vi "诊断标定3 - 副本.vi"(8 "CAN端口":u16(ring), 9 "设备索引号":u16(ring), 10 "CAN卡类型":u32(ring)=21) -> ()   [LabVIEW 2013] (continued)
                    }
                  }
                }
              }
            }
          }
          event "DO1": Value Change {
            n2402 = event-data() -> ("NewVal"=w2943:bool)  [unwired: 6 out]
            n2403 = stacked-sequence {
              tunnel: w2943 -> [_ w2956 _]
              frame #0 {
                w2946 = FALSE ("清BUFF")
                n2404 = local write "继电器超时处理"(FALSE ("继电器超时处理")) -> ()
                n2405 = local write "清BUFF"(w2946) -> ()
                n2406 = local write "正级继电器 9"(w2946) -> ()
                n2407 = local write "主从选择"(enum32{"主板", "从板"}."主板" ("主从选择")) -> ()
              }
              frame #1 {
                n2408 = case shown="真" w2956 {
                  selector: w2956 -> [w2971 w2991]
                  tunnel: [w2970 w2990] -> w2955
                  tunnel: [w2958 w2978] -> w2950
                  frame False {
                    w2966 = 256.0 ("y")
                    w2958 = u32 2 ("命令序号")
                    w2970 = u8 192 ("命令")
                    n2409 = local read "动作保持时间"() -> (w2967:dbl)
                    n2410 = Quotient & Remainder(x=w2967, y=w2966) -> (x-y*floor(x/y)=w2959:dbl, floor(x/y)=w2963:dbl)
                    n2411 = Quotient & Remainder(x=w2963, y=w2966) -> (x-y*floor(x/y)=w2960:dbl, floor(x/y)=w2964:dbl)
                    n2412 = Quotient & Remainder(x=w2964, y=w2966) -> (x-y*floor(x/y)=w2961:dbl, floor(x/y)=w2965:dbl)
                    n2413 = local read "设备索引号"() -> (w2975:u16)
                    n2414 = local read "CAN卡类型"() -> (w2976:u32)
                    n2415 = local read "CAN端口"() -> (w2974:u16)
                    n2416 = Boolean To (0,1)(Boolean=w2971) -> (0, 1=w2968:i16)
                    n2417 = Quotient & Remainder(x=w2965, y=w2966) -> (x-y*floor(x/y)=w2962:dbl)  [unwired: 1 out]
                    n2418 = Build Array(i16 1 ("元素"), w2968, w2962, w2961, w2960, w2959, 0.0 ("元素")) -> (w2972:dbl[])
                    n2419 = call "多帧发送机制(EV05).vi"("can卡类型"=w2976, "设备索引号"=w2975, "CAN端口"=w2974, "命令"=w2970, "板号"=u8 0, "命令序号"=w2958, "输入数据"=w2972) -> ()  [unwired: 1 in, 12 out]
                  }
                  frame True {
                    w2986 = 256.0 ("y")
                    w2978 = u32 2 ("命令序号")
                    w2990 = u8 192 ("命令")
                    n2420 = local read "动作保持时间"() -> (w2987:dbl)
                    n2421 = Quotient & Remainder(x=w2987, y=w2986) -> (x-y*floor(x/y)=w2979:dbl, floor(x/y)=w2983:dbl)
                    n2422 = Quotient & Remainder(x=w2983, y=w2986) -> (x-y*floor(x/y)=w2980:dbl, floor(x/y)=w2984:dbl)
                    n2423 = Quotient & Remainder(x=w2984, y=w2986) -> (x-y*floor(x/y)=w2981:dbl, floor(x/y)=w2985:dbl)
                    n2424 = local read "设备索引号"() -> (w2995:u16)
                    n2425 = local read "CAN卡类型"() -> (w2996:u32)
                    n2426 = local read "CAN端口"() -> (w2994:u16)
                    n2427 = Boolean To (0,1)(Boolean=w2991) -> (0, 1=w2988:i16)
                    n2428 = Quotient & Remainder(x=w2985, y=w2986) -> (x-y*floor(x/y)=w2982:dbl)  [unwired: 1 out]
                    n2429 = Build Array(i16 1 ("元素"), w2988, w2982, w2981, w2980, w2979, 0.0 ("元素")) -> (w2992:dbl[])
                    n2430 = call "多帧发送机制(EV05).vi"("can卡类型"=w2996, "设备索引号"=w2995, "CAN端口"=w2994, "命令"=w2990, "板号"=u8 0, "命令序号"=w2978, "输入数据"=w2992) -> ()  [unwired: 1 in, 12 out]
                  }
                }
                n2431 = local write "命令序号"(w2950) -> ()
                n2432 = local write "命令"(w2955) -> ()
                n2433 = local write "控制1"(TRUE ("控制1")) -> ()
                n2434 = local write "写?"(FALSE ("写?")) -> ()
                n2435 = local write "消除"(TRUE ("消除")) -> ()
                n2436 = global write "EV05全局变量1.vi" "流控帧 2"(TRUE ("流控帧 2")) -> ()
                n2437 = global write "EV05全局变量1.vi" "流控帧"(FALSE ("流控帧")) -> ()
              }
              frame #2 {
                n2438 = flat-sequence {
                  tunnel: [w2998] -> w2997
                  tunnel: w2997 -> [w3005]
                  frame #0 {
                    n2439 = while {
                      tunnel: [w2999] -> w2998
                      i -> [w3003]
                      stop <- w3000 stop-if-true
                      n2440 = local read "继电器超时处理"() -> (w2999:bool)
                      n2441 = Greater Or Equal?(x=w3003, y=20) -> (x >= y?=w3001:bool)
                      n2442 = Wait Until Next ms Multiple(millisecond multiple=u32 100 ("毫秒倍数")) -> ()  [unwired: 1 out]
                      n2443 = Or(x=w2999, y=w3001) -> (x .or. y?=w3000:bool)
                    }
                  }
                  frame #1 {
                    n2444 = case shown="假" w3005 {
                      frame False {
                        n2445 = local read "DO1"() -> (w3007:bool)
                        n2446 = Not(x=w3007) -> (.not. x?=w3006:bool)
                        n2447 = local write "DO1"(w3006) -> ()
                        n2448 = One Button Dialog(message="DO控制处理超时" ("消息"), button name ("OK")="是" ("按钮名称（“确定”）")) -> ()  [unwired: 1 out]
                      }
                      frame True {
                      }
                    }
                  }
                }
              }
            }
          }
          event "DO2": Value Change {
            n2449 = event-data() -> ("NewVal"=w3010:bool)  [unwired: 6 out]
            n2450 = stacked-sequence {
              tunnel: w3010 -> [_ w3023 _]
              frame #0 {
                w3013 = FALSE ("清BUFF")
                n2451 = local write "继电器超时处理"(FALSE ("继电器超时处理")) -> ()
                n2452 = local write "主从选择"(enum32{"主板", "从板"}."主板" ("主从选择")) -> ()
                n2453 = local write "清BUFF"(w3013) -> ()
                n2454 = local write "正级继电器 10"(w3013) -> ()
              }
              frame #1 {
                n2455 = case shown="真" w3023 {
                  selector: w3023 -> [w3038 w3058]
                  tunnel: [w3037 w3057] -> w3022
                  tunnel: [w3025 w3045] -> w3017
                  frame False {
                    w3033 = 256.0 ("y")
                    w3025 = u32 2 ("命令序号")
                    w3037 = u8 192 ("命令")
                    n2456 = local read "动作保持时间"() -> (w3034:dbl)
                    n2457 = Quotient & Remainder(x=w3034, y=w3033) -> (x-y*floor(x/y)=w3026:dbl, floor(x/y)=w3030:dbl)
                    n2458 = Quotient & Remainder(x=w3030, y=w3033) -> (x-y*floor(x/y)=w3027:dbl, floor(x/y)=w3031:dbl)
                    n2459 = Quotient & Remainder(x=w3031, y=w3033) -> (x-y*floor(x/y)=w3028:dbl, floor(x/y)=w3032:dbl)
                    n2460 = local read "设备索引号"() -> (w3042:u16)
                    n2461 = local read "CAN卡类型"() -> (w3043:u32)
                    n2462 = local read "CAN端口"() -> (w3041:u16)
                    n2463 = Boolean To (0,1)(Boolean=w3038) -> (0, 1=w3035:i16)
                    n2464 = Quotient & Remainder(x=w3032, y=w3033) -> (x-y*floor(x/y)=w3029:dbl)  [unwired: 1 out]
                    n2465 = Build Array(i16 2 ("元素"), w3035, w3029, w3028, w3027, w3026, 0.0 ("元素")) -> (w3039:dbl[])
                    n2466 = call "多帧发送机制(EV05).vi"("can卡类型"=w3043, "设备索引号"=w3042, "CAN端口"=w3041, "命令"=w3037, "板号"=u8 0, "命令序号"=w3025, "输入数据"=w3039) -> ()  [unwired: 1 in, 12 out]
                  }
                  frame True {
                    w3053 = 256.0 ("y")
                    w3045 = u32 2 ("命令序号")
                    w3057 = u8 192 ("命令")
                    n2467 = local read "动作保持时间"() -> (w3054:dbl)
                    n2468 = Quotient & Remainder(x=w3054, y=w3053) -> (x-y*floor(x/y)=w3046:dbl, floor(x/y)=w3050:dbl)
                    n2469 = Quotient & Remainder(x=w3050, y=w3053) -> (x-y*floor(x/y)=w3047:dbl, floor(x/y)=w3051:dbl)
                    n2470 = Quotient & Remainder(x=w3051, y=w3053) -> (x-y*floor(x/y)=w3048:dbl, floor(x/y)=w3052:dbl)
                    n2471 = local read "设备索引号"() -> (w3062:u16)
                    n2472 = local read "CAN卡类型"() -> (w3063:u32)
                    n2473 = local read "CAN端口"() -> (w3061:u16)
                    n2474 = Boolean To (0,1)(Boolean=w3058) -> (0, 1=w3055:i16)
                    n2475 = Quotient & Remainder(x=w3052, y=w3053) -> (x-y*floor(x/y)=w3049:dbl)  [unwired: 1 out]
                    n2476 = Build Array(i16 2 ("元素"), w3055, w3049, w3048, w3047, w3046, 0.0 ("元素")) -> (w3059:dbl[])
                    n2477 = call "多帧发送机制(EV05).vi"("can卡类型"=w3063, "设备索引号"=w3062, "CAN端口"=w3061, "命令"=w3057, "板号"=u8 0, "命令序号"=w3045, "输入数据"=w3059) -> ()  [unwired: 1 in, 12 out]
                  }
                }
                n2478 = local write "命令序号"(w3017) -> ()
                n2479 = local write "命令"(w3022) -> ()
                n2480 = local write "控制1"(TRUE ("控制1")) -> ()
                n2481 = local write "写?"(FALSE ("写?")) -> ()
                n2482 = local write "消除"(TRUE ("消除")) -> ()
                n2483 = global write "EV05全局变量1.vi" "流控帧 2"(TRUE ("流控帧 2")) -> ()
                n2484 = global write "EV05全局变量1.vi" "流控帧"(FALSE ("流控帧")) -> ()
              }
              frame #2 {
                n2485 = flat-sequence {
                  tunnel: [w3065] -> w3064
                  tunnel: w3064 -> [w3072]
                  frame #0 {
                    n2486 = while {
                      tunnel: [w3066] -> w3065
                      i -> [w3070]
                      stop <- w3067 stop-if-true
                      n2487 = local read "继电器超时处理"() -> (w3066:bool)
                      n2488 = Greater Or Equal?(x=w3070, y=20) -> (x >= y?=w3068:bool)
                      n2489 = Wait Until Next ms Multiple(millisecond multiple=u32 100 ("毫秒倍数")) -> ()  [unwired: 1 out]
                      n2490 = Or(x=w3066, y=w3068) -> (x .or. y?=w3067:bool)
                    }
                  }
                  frame #1 {
                    n2491 = case shown="假" w3072 {
                      frame False {
                        n2492 = local read "DO2"() -> (w3074:bool)
                        n2493 = Not(x=w3074) -> (.not. x?=w3073:bool)
                        n2494 = local write "DO2"(w3073) -> ()
                        n2495 = One Button Dialog(message="DO控制处理超时" ("消息"), button name ("OK")="是" ("按钮名称（“确定”）")) -> ()  [unwired: 1 out]
                      }
                      frame True {
                      }
                    }
                  }
                }
              }
            }
          }
          event "DO1 2": Value Change {
            n2496 = event-data() -> ("NewVal"=w3077:bool)  [unwired: 6 out]
            n2497 = stacked-sequence {
              tunnel: w3077 -> [_ w3091 _]
              frame #0 {
                w3080 = FALSE ("继电器超时处理")
                n2498 = local write "继电器超时处理"(w3080) -> ()
                n2499 = local write "正级继电器 11"(w3080) -> ()
                n2500 = local write "主从选择"(enum32{"主板", "从板"}."从板" ("主从选择")) -> ()
              }
              frame #1 {
                n2501 = case shown="假" w3091 {
                  selector: w3091 -> [w3106 w3126]
                  tunnel: [w3105 w3125] -> w3090
                  tunnel: [w3104 w3124] -> w3084
                  tunnel: [w3093 w3113] -> w3085
                  frame True {
                    w3101 = 256.0 ("y")
                    w3093 = u32 2 ("命令序号")
                    w3105 = u8 192 ("命令")
                    n2502 = local read "动作保持时间"() -> (w3102:dbl)
                    n2503 = Quotient & Remainder(x=w3102, y=w3101) -> (x-y*floor(x/y)=w3094:dbl, floor(x/y)=w3098:dbl)
                    n2504 = Quotient & Remainder(x=w3098, y=w3101) -> (x-y*floor(x/y)=w3095:dbl, floor(x/y)=w3099:dbl)
                    n2505 = Quotient & Remainder(x=w3099, y=w3101) -> (x-y*floor(x/y)=w3096:dbl, floor(x/y)=w3100:dbl)
                    n2506 = Quotient & Remainder(x=w3100, y=w3101) -> (x-y*floor(x/y)=w3097:dbl)  [unwired: 1 out]
                    n2507 = Boolean To (0,1)(Boolean=w3106) -> (0, 1=w3103:i16)
                    n2508 = local read "设备索引号"() -> (w3110:u16)
                    n2509 = local read "CAN卡类型"() -> (w3111:u32)
                    n2510 = local read "从板板号"() -> (w3104:u8)
                    n2511 = local read "CAN端口"() -> (w3109:u16)
                    n2512 = Build Array(i16 3 ("元素"), w3103, w3097, w3096, w3095, w3094, 0.0 ("元素")) -> (w3108:dbl[])
                    n2513 = call "多帧发送机制(EV05).vi"("can卡类型"=w3111, "设备索引号"=w3110, "CAN端口"=w3109, "命令"=w3105, "板号"=w3104, "命令序号"=w3093, "输入数据"=w3108) -> ()  [unwired: 1 in, 12 out]
                  }
                  frame False {
                    w3121 = 256.0 ("y")
                    w3113 = u32 2 ("命令序号")
                    w3125 = u8 192 ("命令")
                    n2514 = local read "动作保持时间"() -> (w3122:dbl)
                    n2515 = Quotient & Remainder(x=w3122, y=w3121) -> (x-y*floor(x/y)=w3114:dbl, floor(x/y)=w3118:dbl)
                    n2516 = Quotient & Remainder(x=w3118, y=w3121) -> (x-y*floor(x/y)=w3115:dbl, floor(x/y)=w3119:dbl)
                    n2517 = Quotient & Remainder(x=w3119, y=w3121) -> (x-y*floor(x/y)=w3116:dbl, floor(x/y)=w3120:dbl)
                    n2518 = Quotient & Remainder(x=w3120, y=w3121) -> (x-y*floor(x/y)=w3117:dbl)  [unwired: 1 out]
                    n2519 = Boolean To (0,1)(Boolean=w3126) -> (0, 1=w3123:i16)
                    n2520 = local read "设备索引号"() -> (w3130:u16)
                    n2521 = local read "CAN卡类型"() -> (w3131:u32)
                    n2522 = local read "从板板号"() -> (w3124:u8)
                    n2523 = local read "CAN端口"() -> (w3129:u16)
                    n2524 = Build Array(i16 1 ("元素"), w3123, w3117, w3116, w3115, w3114, 0.0 ("元素")) -> (w3128:dbl[])
                    n2525 = call "多帧发送机制(EV05).vi"("can卡类型"=w3131, "设备索引号"=w3130, "CAN端口"=w3129, "命令"=w3125, "板号"=w3124, "命令序号"=w3113, "输入数据"=w3128) -> ()  [unwired: 1 in, 12 out]
                  }
                }
                n2526 = local write "从板板号"(w3084) -> ()
                n2527 = local write "命令序号"(w3085) -> ()
                n2528 = local write "命令"(w3090) -> ()
                n2529 = local write "清BUFF"(FALSE ("清BUFF")) -> ()
                n2530 = local write "写?"(FALSE ("写?")) -> ()
                n2531 = local write "控制1"(TRUE ("控制1")) -> ()
                n2532 = global write "EV05全局变量1.vi" "流控帧"(FALSE ("流控帧")) -> ()
                n2533 = global write "EV05全局变量1.vi" "流控帧 2"(TRUE ("流控帧 2")) -> ()
                n2534 = local write "消除"(TRUE ("消除")) -> ()
              }
              frame #2 {
                n2535 = flat-sequence {
                  tunnel: [w3133] -> w3132
                  tunnel: w3132 -> [w3140]
                  frame #0 {
                    n2536 = while {
                      tunnel: [w3134] -> w3133
                      i -> [w3138]
                      stop <- w3135 stop-if-true
                      n2537 = local read "继电器超时处理"() -> (w3134:bool)
                      n2538 = Greater Or Equal?(x=w3138, y=20) -> (x >= y?=w3136:bool)
                      n2539 = Wait Until Next ms Multiple(millisecond multiple=u32 100 ("毫秒倍数")) -> ()  [unwired: 1 out]
                      n2540 = Or(x=w3134, y=w3136) -> (x .or. y?=w3135:bool)
                    }
                  }
                  frame #1 {
                    n2541 = case shown="假" w3140 {
                      frame False {
                        n2542 = local read "DO1 2"() -> (w3142:bool)
                        n2543 = Not(x=w3142) -> (.not. x?=w3141:bool)
                        n2544 = local write "DO1 2"(w3141) -> ()
                        n2545 = One Button Dialog(message="DO控制处理超时" ("消息"), button name ("OK")="是" ("按钮名称（“确定”）")) -> ()  [unwired: 1 out]
                      }
                      frame True {
                      }
                    }
                  }
                }
              }
            }
          }
          event "读取转换为写入": Value Change {
            n2546 = event-data() -> ("NewVal"=w3145:bool)  [unwired: 6 out]
            n2547 = case shown="真" w3145 {
              tunnel: w3149 -> [w3151 w3156]
              tunnel: [w3151 w3155] -> w3148
              tunnel: w3147 -> [w3150 w3154]
              tunnel: [w3150 w3153] -> w3146
              frame False {
              }
              frame True {
                n2548 = Enqueue Element(queue=w3156, element="读取转换为写入", error in (no error)=w3154) -> (queue out=w3155:refnum<queue>, error out=w3153:errorcluster)  [unwired: 2 out]
              }
            }
          }
          event "读取故障详细状态": Value Change {
            n2549 = event-data() -> ("NewVal"=w3161:bool)  [unwired: 5 out]
            n2550 = case shown="真" w3161 {
              tunnel: w3160 -> [w3163 w3176]
              tunnel: w3159 -> [w3162 w3175]
              tunnel: [w3163 w3174] -> w3158
              tunnel: [w3162 w3173] -> w3157
              frame False {
              }
              frame True {
                n2551 = disable-structure shown="启用" {
                  disable-tunnel: [w3185 TRUE ("发送成功")] -> w3172
                  frame Disabled {
                    n2552 = local read "主从选择"() -> (w3177:enum32{"主板", "从板"})
                    n2553 = case shown="\"主板\", 默认" w3177 {
                      tunnel: [0.0 ("FUNC") w3187] -> w3182
                      frame "主板", Default {
                      }
                      frame "从板" {
                        n2554 = local read "从板号"() -> (w3187:u8)
                      }
                    }
                    n2555 = local read "设备索引号"() -> (w3179:u16)
                    n2556 = local read "CAN卡类型"() -> (w3180:u32)
                    n2557 = local read "CAN端口"() -> (w3178:u16)
                    n2558 = call "标定授权发送.vi"("CAN卡类型"=w3180, "解锁类型"=enum16{"读取", "写", "下载"}."写", "设备索引号"=w3179, "CAN端口"=w3178, "是否连接"=TRUE, "板选择"=0, "FUNC"=w3182) -> ("发送成功"=w3185:bool)  [unwired: 8 out]
                  }
                  frame Enabled {
                  }
                }
                n2559 = case shown="真" w3172 {
                  tunnel: w3176 -> [w3190 w3195]
                  tunnel: w3175 -> [w3189 w3194]
                  tunnel: [w3190 w3192] -> w3174
                  tunnel: [w3189 w3191] -> w3173
                  frame False {
                  }
                  frame True {
                    n2560 = Enqueue Element(queue=w3195, element="读取故障状态" ("元素"), error in (no error)=w3194) -> (queue out=w3192:refnum<queue>, error out=w3191:errorcluster)  [unwired: 2 out]
                  }
                }
                n2561 = local write "电池故障"(string[][] []) -> ()
                n2562 = global write "EV05全局变量1.vi" "流控帧 2"(TRUE ("流控帧")) -> ()
                n2563 = local write "写?"(FALSE ("写?")) -> ()
                n2564 = local write "控制1"(TRUE ("控制1")) -> ()
                n2565 = local write "消除"(TRUE ("消除")) -> ()
                n2566 = local write "清BUFF"(FALSE ("清BUFF")) -> ()
                n2567 = global write "EV05全局变量1.vi" "流控帧"(FALSE ("流控帧")) -> ()
                n2568 = call <vilib>:"Set Busy.vi"("disable click? (T)"=FALSE) -> ()  [unwired: 3 in, 8 out]
              }
            }
          }
          event "项目软本读取": Value Change {
            n2569 = event-data() -> ("NewVal"=w3200:bool)  [unwired: 5 out]
            n2570 = case shown="真" w3200 {
              tunnel: w3199 -> [w3202 w3209]
              tunnel: w3198 -> [w3201 w3208]
              tunnel: [w3202 w3207] -> w3197
              tunnel: [w3201 w3206] -> w3196
              frame False {
              }
              frame True {
                n2571 = global read "EV05全局变量1.vi" "授权功能"() -> (w3204:bool)
                n2572 = case shown="假" w3204 {
                  tunnel: [TRUE ("发送成功") w3228] -> w3205
                  frame False {
                  }
                  frame True {
                    n2573 = local read "设备索引号"() -> (w3223:u16)
                    n2574 = local read "CAN卡类型"() -> (w3224:u32)
                    n2575 = local read "CAN端口"() -> (w3222:u16)
                    n2576 = call "标定授权发送.vi"("CAN卡类型"=w3224, "解锁类型"=enum16{"读取", "写", "下载"}."读取", "设备索引号"=w3223, "CAN端口"=w3222, "是否连接"=TRUE, "板选择"=0, "FUNC"=u32 0) -> ("发送成功"=w3228:bool)  [unwired: 8 out]
                  }
                }
                n2577 = stacked-sequence {
                  tunnel: [w3212] -> w3203
                  frame #0 {
                    w3212 = FALSE ("disable click? (T)")
                    w3215 = FALSE ("写?")
                    n2578 = local write "写?"(w3215) -> ()
                    n2579 = global write "EV05全局变量1.vi" "写入超时"(w3215) -> ()
                    n2580 = local write "项目软件版本号"(" " ("项目软件版本号")) -> ()
                    n2581 = global write "EV05全局变量1.vi" "流控帧"(FALSE ("流控帧")) -> ()
                    n2582 = local write "主从选择"(enum32{"主板", "从板"}."主板" ("主从选择")) -> ()
                    n2583 = call <vilib>:"Set Busy.vi"("disable click? (T)"=w3212) -> ()  [unwired: 3 in, 8 out]
                    n2584 = local write "清BUFF"(FALSE ("清BUFF")) -> ()
                    n2585 = property on="保存版本信息" class="Bool (严格)"("Visible"=TRUE ("可见")) -> ()  [unwired: 2 in, 2 out]
                    n2586 = global write "EV05全局变量1.vi" "流控帧 2"(TRUE ("流控帧 2")) -> ()
                    n2587 = local write "控制1"(TRUE ("控制1")) -> ()
                    n2588 = local write "消除"(TRUE ("消除")) -> ()
                  }
                }
                n2589 = case shown="真" w3205 {
                  tunnel: w3209 -> [w3230 w3235]
                  tunnel: w3208 -> [w3229 w3234]
                  tunnel: [w3230 w3232] -> w3207
                  tunnel: [w3229 w3231] -> w3206
                  tunnel: w3203 -> [_ _]
                  frame False {
                  }
                  frame True {
                    n2590 = Enqueue Element(queue=w3235, element="项目软件版本读取" ("元素"), error in (no error)=w3234) -> (queue out=w3232:refnum<queue>, error out=w3231:errorcluster)  [unwired: 2 out]
                  }
                }
              }
            }
          }
          event "读硬件版本号": Value Change {
            n2591 = event-data() -> ("NewVal"=w3240:bool)  [unwired: 5 out]
            n2592 = case shown="真" w3240 {
              tunnel: w3239 -> [w3242 w3249]
              tunnel: w3238 -> [w3241 w3248]
              tunnel: [w3242 w3247] -> w3237
              tunnel: [w3241 w3246] -> w3236
              frame False {
              }
              frame True {
                n2593 = global read "EV05全局变量1.vi" "授权功能"() -> (w3244:bool)
                n2594 = case shown="假" w3244 {
                  tunnel: [TRUE ("发送成功") w3268] -> w3245
                  frame False {
                  }
                  frame True {
                    n2595 = local read "设备索引号"() -> (w3263:u16)
                    n2596 = local read "CAN卡类型"() -> (w3264:u32)
                    n2597 = local read "CAN端口"() -> (w3262:u16)
                    n2598 = call "标定授权发送.vi"("CAN卡类型"=w3264, "解锁类型"=enum16{"读取", "写", "下载"}."读取", "设备索引号"=w3263, "CAN端口"=w3262, "是否连接"=TRUE, "板选择"=0, "FUNC"=u32 0) -> ("发送成功"=w3268:bool)  [unwired: 8 out]
                  }
                }
                n2599 = stacked-sequence {
                  tunnel: [w3252] -> w3243
                  frame #0 {
                    w3252 = TRUE ("控制1")
                    w3256 = FALSE ("写?")
                    n2600 = local write "写?"(w3256) -> ()
                    n2601 = global write "EV05全局变量1.vi" "写入超时"(w3256) -> ()
                    n2602 = call <vilib>:"Set Busy.vi"("disable click? (T)"=FALSE) -> ()  [unwired: 3 in, 8 out]
                    n2603 = local write "硬件版本号"("" ("硬件版本号")) -> ()
                    n2604 = property on="保存版本信息" class="Bool (严格)"("Visible"=TRUE ("可见")) -> ()  [unwired: 2 in, 2 out]
                    n2605 = local write "主从选择"(enum32{"主板", "从板"}."主板" ("主从选择")) -> ()
                    n2606 = local write "控制1"(w3252) -> ()
                    n2607 = local write "清BUFF"(FALSE ("清BUFF")) -> ()
                    n2608 = global write "EV05全局变量1.vi" "流控帧 2"(TRUE ("流控帧 2")) -> ()
                    n2609 = local write "消除"(TRUE ("消除")) -> ()
                    n2610 = global write "EV05全局变量1.vi" "流控帧"(FALSE ("流控帧")) -> ()
                  }
                }
                n2611 = case shown="真" w3245 {
                  tunnel: w3249 -> [w3270 w3275]
                  tunnel: w3248 -> [w3269 w3274]
                  tunnel: [w3270 w3272] -> w3247
                  tunnel: [w3269 w3271] -> w3246
                  tunnel: w3243 -> [_ _]
                  frame False {
                  }
                  frame True {
                    n2612 = Enqueue Element(queue=w3275, element="硬件版本读取" ("元素"), error in (no error)=w3274) -> (queue out=w3272:refnum<queue>, error out=w3271:errorcluster)  [unwired: 2 out]
                  }
                }
              }
            }
          }
          event "平台软件版本读取": Value Change {
            n2613 = event-data() -> ("NewVal"=w3280:bool)  [unwired: 5 out]
            n2614 = case shown="真" w3280 {
              tunnel: w3279 -> [w3282 w3289]
              tunnel: w3278 -> [w3281 w3288]
              tunnel: [w3282 w3287] -> w3277
              tunnel: [w3281 w3286] -> w3276
              frame False {
              }
              frame True {
                n2615 = global read "EV05全局变量1.vi" "授权功能"() -> (w3284:bool)
                n2616 = case shown="假" w3284 {
                  tunnel: [TRUE ("发送成功") w3308] -> w3285
                  frame False {
                  }
                  frame True {
                    n2617 = local read "设备索引号"() -> (w3303:u16)
                    n2618 = local read "CAN卡类型"() -> (w3304:u32)
                    n2619 = local read "CAN端口"() -> (w3302:u16)
                    n2620 = call "标定授权发送.vi"("CAN卡类型"=w3304, "解锁类型"=enum16{"读取", "写", "下载"}."读取", "设备索引号"=w3303, "CAN端口"=w3302, "是否连接"=TRUE, "板选择"=0, "FUNC"=u32 0) -> ("发送成功"=w3308:bool)  [unwired: 8 out]
                  }
                }
                n2621 = stacked-sequence {
                  tunnel: [w3292] -> w3283
                  frame #0 {
                    w3292 = TRUE ("控制1")
                    w3296 = FALSE ("写?")
                    n2622 = call <vilib>:"Set Busy.vi"("disable click? (T)"=FALSE) -> ()  [unwired: 3 in, 8 out]
                    n2623 = local write "写?"(w3296) -> ()
                    n2624 = global write "EV05全局变量1.vi" "写入超时"(w3296) -> ()
                    n2625 = local write "平台软件版本号"(" " ("平台软件版本号")) -> ()
                    n2626 = local write "控制1"(w3292) -> ()
                    n2627 = local write "消除"(TRUE ("消除")) -> ()
                    n2628 = property on="保存版本信息" class="Bool (严格)"("Visible"=TRUE ("可见")) -> ()  [unwired: 2 in, 2 out]
                    n2629 = global write "EV05全局变量1.vi" "流控帧 2"(TRUE ("流控帧 2")) -> ()
                    n2630 = local write "主从选择"(enum32{"主板", "从板"}."主板" ("主从选择")) -> ()
                    n2631 = local write "清BUFF"(FALSE ("清BUFF")) -> ()
                    n2632 = global write "EV05全局变量1.vi" "流控帧"(FALSE ("流控帧")) -> ()
                  }
                }
                n2633 = case shown="真" w3285 {
                  tunnel: w3289 -> [w3310 w3315]
                  tunnel: w3288 -> [w3309 w3314]
                  tunnel: [w3310 w3312] -> w3287
                  tunnel: [w3309 w3311] -> w3286
                  tunnel: w3283 -> [_ _]
                  frame False {
                  }
                  frame True {
                    n2634 = Enqueue Element(queue=w3315, element="平台软件版本读取" ("元素"), error in (no error)=w3314) -> (queue out=w3312:refnum<queue>, error out=w3311:errorcluster)  [unwired: 2 out]
                  }
                }
              }
            }
          }
          event "模块版本读取": Value Change {
            n2635 = event-data() -> ("NewVal"=w3320:bool)  [unwired: 5 out]
            n2636 = case shown="真" w3320 {
              tunnel: w3319 -> [w3322 w3329]
              tunnel: w3318 -> [w3321 w3328]
              tunnel: [w3322 w3327] -> w3317
              tunnel: [w3321 w3326] -> w3316
              frame False {
              }
              frame True {
                n2637 = global read "EV05全局变量1.vi" "授权功能"() -> (w3324:bool)
                n2638 = case shown="假" w3324 {
                  tunnel: [TRUE ("发送成功") w3347] -> w3325
                  frame False {
                  }
                  frame True {
                    n2639 = local read "设备索引号"() -> (w3342:u16)
                    n2640 = local read "CAN卡类型"() -> (w3343:u32)
                    n2641 = local read "CAN端口"() -> (w3341:u16)
                    n2642 = call "标定授权发送.vi"("CAN卡类型"=w3343, "解锁类型"=enum16{"读取", "写", "下载"}."读取", "设备索引号"=w3342, "CAN端口"=w3341, "是否连接"=TRUE, "板选择"=0, "FUNC"=u32 0) -> ("发送成功"=w3347:bool)  [unwired: 8 out]
                  }
                }
                n2643 = stacked-sequence {
                  tunnel: [w3332] -> w3323
                  frame #0 {
                    w3332 = TRUE ("控制1")
                    w3335 = FALSE ("写?")
                    n2644 = call <vilib>:"Set Busy.vi"("disable click? (T)"=FALSE) -> ()  [unwired: 3 in, 8 out]
                    n2645 = local write "写?"(w3335) -> ()
                    n2646 = global write "EV05全局变量1.vi" "写入超时"(w3335) -> ()
                    n2647 = local write "主从选择"(enum32{"主板", "从板"}."主板" ("主从选择")) -> ()
                    n2648 = local write "清BUFF"(FALSE ("清BUFF")) -> ()
                    n2649 = property on="保存版本信息" class="Bool (严格)"("Visible"=TRUE ("可见")) -> ()  [unwired: 2 in, 2 out]
                    n2650 = global write "EV05全局变量1.vi" "流控帧 2"(TRUE ("流控帧 2")) -> ()
                    n2651 = local write "控制1"(w3332) -> ()
                    n2652 = local write "消除"(TRUE ("消除")) -> ()
                    n2653 = global write "EV05全局变量1.vi" "流控帧"(FALSE ("流控帧")) -> ()
                  }
                }
                n2654 = case shown="真" w3325 {
                  tunnel: w3329 -> [w3349 w3354]
                  tunnel: w3328 -> [w3348 w3353]
                  tunnel: [w3349 w3351] -> w3327
                  tunnel: [w3348 w3350] -> w3326
                  tunnel: w3323 -> [_ _]
                  frame False {
                  }
                  frame True {
                    n2655 = Enqueue Element(queue=w3354, element="模块软件版本读取" ("元素"), error in (no error)=w3353) -> (queue out=w3351:refnum<queue>, error out=w3350:errorcluster)  [unwired: 2 out]
                  }
                }
              }
            }
          }
          event "保存版本信息": Value Change {
            n2656 = event-data() -> ("NewVal"=w3355:bool)  [unwired: 6 out]
            n2657 = case shown="真" w3355 {
              frame False {
              }
              frame True {
                n2658 = stacked-sequence {
                  seq-local: [w3359 _] -> [_ w3361]
                  seq-local: [w3358 _] -> [_ w3360]
                  frame #0 {
                    n2659 = call "请输入从板个数"() -> ("从板个数"=w3359:dbl, "确定"=w3358:bool)  [unwired: 17 in, 1 out]
                  }
                  frame #1 {
                    n2660 = case shown="真" w3360 {
                      tunnel: w3361 -> [_ w3364]
                      frame False {
                      }
                      frame True {
                        n2661 = call <vilib>:"Application Directory.vi"() -> ("Application Directory"=w3376:path)
                        n2662 = Build Path(base path=w3376, name or relative path="SaveData" ("名称或相对路径")) -> (appended path=w3374:path)
                        n2663 = local read "模块版本名称"() -> (w3369:string[][])
                        n2664 = local read "项目软件版本"() -> (w3366:string[])
                        n2665 = local read "模块版本值"() -> (w3368:string[][])
                        n2666 = local read "平台软件版本"() -> (w3365:string[])
                        n2667 = local read "模块个数"() -> (w3362:u8[])
                        n2668 = local read "硬件版本"() -> (w3367:string[])
                        n2669 = call "文件对话框3"("start path"=w3374, "prompt"="选择要保存数据的位置", "default name"="BMS版本信息.txt") -> ("selected path"=w3370:path, "cancelled"=w3371:bool)  [unwired: 9 in, 2 out]
                        n2670 = Increment(x=w3364) -> (x+1=w3363:dbl)
                        n2671 = for {
                          N: w3363 -> [_]
                          tunnel: w3371 -> [w3392]
                          tunnel: w3370 -> [w3391]
                          tunnel: w3369 -> [w3381] mode=indexing
                          tunnel: w3368 -> [w3379] mode=indexing
                          tunnel: w3367 -> [w3386] mode=indexing
                          tunnel: w3366 -> [w3385] mode=indexing
                          tunnel: w3365 -> [w3384] mode=indexing
                          tunnel: w3362 -> [w3377] mode=indexing
                          i -> [w3383]
                          w3389 = ""
                          w3396 = 0 ("索引")
                          n2672 = case shown="0, 默认" w3383 {
                            selector: w3383 -> [_ w3410]
                            tunnel: ["主板版本信息" w3411] -> w3401
                            tunnel: [FALSE TRUE] -> w3387
                            frame 0, Default {
                            }
                            frame 1.. {
                              n2673 = Number To Decimal String(number=w3410) -> (decimal integer string=w3409:string)  [unwired: 1 in]
                              n2674 = Concatenate Strings("从板", w3409, "版本信息") -> (w3411:string)
                            }
                          }
                          n2675 = Increment(x=w3377) -> (x+1=w3378:u8)
                          n2676 = Array Subset(array=w3381, length=w3378) -> (w3382:string[])  [unwired: 1 in]
                          n2677 = Array Subset(array=w3379, length=w3378) -> (w3380:string[])  [unwired: 1 in]
                          n2678 = Build Array(w3389, w3384, w3385, w3386, w3389) -> (w3395:string[])
                          n2679 = Build Array(w3401, "平台软件版本号", "项目软件版本号", "硬件版本号", "模块版本号") -> (w3397:string[])
                          n2680 = Insert Into Array(array=w3382, index=w3396, new element=w3397) -> (w3394:string[])
                          n2681 = Insert Into Array(array=w3380, index=w3396, new element=w3395) -> (w3393:string[])
                          n2682 = Build Array(w3394, w3393) -> (w3390:string[][])
                          n2683 = case shown="假" w3392 {
                            tunnel: w3391 -> [w3405 _]
                            tunnel: w3390 -> [w3404 _]
                            tunnel: w3387 -> [w3402 _]
                            frame False {
                              n2684 = call-poly <vilib>:"Write To Spreadsheet File.vi"("transpose? (no:F)"=TRUE, "append to file? (new file:F)"=w3402, "2D data"=w3404, "file path (dialog if empty)"=w3405) -> ()  [unwired: 4 in, 1 out]
                            }
                            frame True {
                            }
                          }
                        }
                      }
                    }
                  }
                }
              }
            }
          }
          event "单个写入": Value Change {
            n2685 = event-data() -> ("NewVal"=w3418:bool)  [unwired: 5 out]
            n2686 = case shown="真" w3418 {
              tunnel: w3417 -> [w3420 w3427]
              tunnel: w3416 -> [w3419 w3426]
              tunnel: [w3420 w3425] -> w3415
              tunnel: [w3419 w3424] -> w3414
              frame False {
              }
              frame True {
                w3422 = FALSE ("流控帧")
                w3421 = TRUE ("流控帧 2")
                n2687 = disable-structure shown="启用" {
                  disable-tunnel: [w3436 TRUE ("发送成功")] -> w3423
                  frame Disabled {
                    n2688 = local read "主从选择"() -> (w3428:enum32{"主板", "从板"})
                    n2689 = case shown="\"主板\", 默认" w3428 {
                      tunnel: [0.0 ("FUNC") w3438] -> w3433
                      frame "主板", Default {
                      }
                      frame "从板" {
                        n2690 = local read "从板号"() -> (w3438:u8)
                      }
                    }
                    n2691 = local read "设备索引号"() -> (w3430:u16)
                    n2692 = local read "CAN卡类型"() -> (w3431:u32)
                    n2693 = local read "CAN端口"() -> (w3429:u16)
                    n2694 = call "标定授权发送.vi"("CAN卡类型"=w3431, "解锁类型"=enum16{"读取", "写", "下载"}."写", "设备索引号"=w3430, "CAN端口"=w3429, "是否连接"=TRUE, "板选择"=0, "FUNC"=w3433) -> ("发送成功"=w3436:bool)  [unwired: 8 out]
                  }
                  frame Enabled {
                  }
                }
                n2695 = case shown="真" w3423 {
                  tunnel: w3427 -> [w3441 w3445]
                  tunnel: w3426 -> [w3440 w3444]
                  tunnel: [w3441 w3447] -> w3425
                  tunnel: [w3440 w3446] -> w3424
                  frame False {
                  }
                  frame True {
                    n2696 = Flush Queue(queue=w3445, error in (no error)=w3444) -> (queue out=w3443:refnum<queue>, error out=w3442:errorcluster)  [unwired: 1 out]
                    n2697 = Enqueue Element(queue=w3443, element="单个写入" ("元素"), error in (no error)=w3442) -> (queue out=w3447:refnum<queue>, error out=w3446:errorcluster)  [unwired: 2 out]
                  }
                }
                n2698 = global write "EV05全局变量1.vi" "读取超时"(w3422) -> ()
                n2699 = global write "EV05全局变量1.vi" "流控帧"(w3422) -> ()
                n2700 = local write "消除"(w3421) -> ()
                n2701 = local write "控制1"(w3421) -> ()
                n2702 = global write "EV05全局变量1.vi" "流控帧 2"(w3421) -> ()
                n2703 = local write "写?"(w3421) -> ()
              }
            }
          }
          event "全部写入": Value Change {
            n2704 = event-data() -> ("NewVal"=w3453:bool)  [unwired: 5 out]
            n2705 = case shown="真" w3453 {
              tunnel: w3452 -> [w3455 w3463]
              tunnel: w3451 -> [w3454 w3462]
              tunnel: [w3455 w3461] -> w3450
              tunnel: [w3454 w3460] -> w3449
              frame False {
              }
              frame True {
                w3457 = FALSE ("流控帧")
                w3456 = TRUE ("流控帧 2")
                n2706 = global read "EV05全局变量1.vi" "授权功能"() -> (w3458:bool)
                n2707 = case shown="真" w3458 {
                  tunnel: [TRUE ("发送成功") w3473] -> w3459
                  frame False {
                  }
                  frame True {
                    n2708 = local read "主从选择"() -> (w3465:enum32{"主板", "从板"})
                    n2709 = case shown="\"从板\"" w3465 {
                      tunnel: [0.0 ("FUNC") w3475] -> w3466
                      frame "主板", Default {
                      }
                      frame "从板" {
                        n2710 = local read "从板号"() -> (w3475:u8)
                      }
                    }
                    n2711 = local read "设备索引号"() -> (w3468:u16)
                    n2712 = local read "CAN卡类型"() -> (w3469:u32)
                    n2713 = local read "CAN端口"() -> (w3467:u16)
                    n2714 = call "标定授权发送.vi"("CAN卡类型"=w3469, "解锁类型"=enum16{"读取", "写", "下载"}."写", "设备索引号"=w3468, "CAN端口"=w3467, "是否连接"=TRUE, "板选择"=0, "FUNC"=w3466) -> ("发送成功"=w3473:bool)  [unwired: 8 out]
                  }
                }
                n2715 = case shown="真" w3459 {
                  tunnel: w3463 -> [w3477 w3481]
                  tunnel: w3462 -> [w3476 w3480]
                  tunnel: [w3477 w3483] -> w3461
                  tunnel: [w3476 w3482] -> w3460
                  frame False {
                  }
                  frame True {
                    n2716 = Flush Queue(queue=w3481, error in (no error)=w3480) -> (queue out=w3479:refnum<queue>, error out=w3478:errorcluster)  [unwired: 1 out]
                    n2717 = Enqueue Element(queue=w3479, element="全部写入" ("元素"), error in (no error)=w3478) -> (queue out=w3483:refnum<queue>, error out=w3482:errorcluster)  [unwired: 1 in, 1 out]
                  }
                }
                n2718 = global write "EV05全局变量1.vi" "读取超时"(w3457) -> ()
                n2719 = global write "EV05全局变量1.vi" "流控帧"(w3457) -> ()
                n2720 = local write "消除"(w3456) -> ()
                n2721 = local write "控制1"(w3456) -> ()
                n2722 = global write "EV05全局变量1.vi" "流控帧 2"(w3456) -> ()
                n2723 = local write "写?"(w3456) -> ()
              }
            }
          }
          event "单个读取": Value Change {
            n2724 = event-data() -> ("NewVal"=w3489:bool)  [unwired: 5 out]
            n2725 = case shown="真" w3489 {
              tunnel: w3488 -> [w3491 w3499]
              tunnel: w3487 -> [w3490 w3498]
              tunnel: [w3491 w3497] -> w3486
              tunnel: [w3490 w3496] -> w3485
              frame False {
              }
              frame True {
                w3492 = FALSE ("流控帧")
                w3493 = TRUE ("流控帧 2")
                n2726 = global read "EV05全局变量1.vi" "授权功能"() -> (w3494:bool)
                n2727 = case shown="假" w3494 {
                  tunnel: [TRUE ("发送成功") w3508] -> w3495
                  frame False {
                  }
                  frame True {
                    n2728 = local read "设备索引号"() -> (w3502:u16)
                    n2729 = local read "CAN卡类型"() -> (w3503:u32)
                    n2730 = local read "CAN端口"() -> (w3501:u16)
                    n2731 = call "标定授权发送.vi"("CAN卡类型"=w3503, "解锁类型"=enum16{"读取", "写", "下载"}."读取", "设备索引号"=w3502, "CAN端口"=w3501, "是否连接"=TRUE, "板选择"=0, "FUNC"=u32 1) -> ("发送成功"=w3508:bool)  [unwired: 8 out]
                  }
                }
                n2732 = case shown="真" w3495 {
                  tunnel: w3499 -> [w3510 w3514]
                  tunnel: w3498 -> [w3509 w3512]
                  tunnel: [w3510 w3516] -> w3497
                  tunnel: [w3509 w3515] -> w3496
                  frame False {
                  }
                  frame True {
                    n2733 = Flush Queue(queue=w3514, error in (no error)=w3512) -> (queue out=w3513:refnum<queue>, error out=w3511:errorcluster)  [unwired: 1 out]
                    n2734 = Enqueue Element(queue=w3513, element="单个读取" ("元素"), error in (no error)=w3511) -> (queue out=w3516:refnum<queue>, error out=w3515:errorcluster)  [unwired: 2 out]
                  }
                }
                n2735 = global write "EV05全局变量1.vi" "写入超时"(w3492) -> ()
                n2736 = global write "EV05全局变量1.vi" "流控帧"(w3492) -> ()
                n2737 = local write "写?"(w3492) -> ()
                n2738 = local write "消除"(w3493) -> ()
                n2739 = local write "控制1"(w3493) -> ()
                n2740 = global write "EV05全局变量1.vi" "流控帧 2"(w3493) -> ()
              }
            }
          }
          event "全部读取": Value Change {
            n2741 = event-data() -> ("NewVal"=w3522:bool)  [unwired: 5 out]
            n2742 = case shown="真" w3522 {
              tunnel: w3521 -> [w3524 w3528]
              tunnel: w3520 -> [w3523 w3527]
              tunnel: [w3524 w3526] -> w3519
              tunnel: [w3523 w3525] -> w3518
              frame False {
              }
              frame True {
                n2743 = stacked-sequence {
                  seq-local: [w3533 _] -> [_ _]
                  seq-local: [w3532 _] -> [_ _]
                  tunnel: w3528 -> [w3535 w3565]
                  tunnel: w3527 -> [w3534 w3564]
                  tunnel: [_ w3569] -> w3526
                  tunnel: [_ w3568] -> w3525
                  frame #0 {
                    w3529 = FALSE ("布尔")
                    n2744 = local read "路径"() -> (w3531:path)
                    n2745 = Empty String/Path?(string/path=w3531) -> (empty?=w3530:bool)
                    n2746 = case shown="假" w3530 {
                      tunnel: w3535 -> [w3543 w3561]
                      tunnel: w3534 -> [w3542 w3560]
                      tunnel: [w3539 w3560] -> w3533
                      tunnel: [w3538 w3561] -> w3532
                      frame False {
                        n2747 = global read "EV05全局变量1.vi" "授权功能"() -> (w3540:bool)
                        n2748 = case shown="真" w3540 {
                          tunnel: [TRUE ("发送成功") w3552] -> w3541
                          frame False {
                          }
                          frame True {
                            n2749 = local read "设备索引号"() -> (w3546:u16)
                            n2750 = local read "CAN卡类型"() -> (w3547:u32)
                            n2751 = local read "CAN端口"() -> (w3545:u16)
                            n2752 = call "标定授权发送.vi"("CAN卡类型"=w3547, "解锁类型"=enum16{"读取", "写", "下载"}."读取", "设备索引号"=w3546, "CAN端口"=w3545, "是否连接"=TRUE, "板选择"=0, "FUNC"=u32 1) -> ("发送成功"=w3552:bool)  [unwired: 8 out]
                          }
                        }
                        n2753 = case shown="真" w3541 {
                          tunnel: w3543 -> [w3554 w3559]
                          tunnel: w3542 -> [w3553 w3558]
                          tunnel: [w3554 w3556] -> w3538
                          tunnel: [w3553 w3555] -> w3539
                          frame False {
                          }
                          frame True {
                            n2754 = Enqueue Element(queue=w3559, element="读配置文件" ("元素"), error in (no error)=w3558) -> (queue out=w3556:refnum<queue>, error out=w3555:errorcluster)  [unwired: 2 out]
                          }
                        }
                        n2755 = local write "布尔"(FALSE ("布尔")) -> ()
                        n2756 = Wait Until Next ms Multiple(millisecond multiple=u32 200 ("毫秒倍数")) -> ()  [unwired: 1 out]
                      }
                      frame True {
                      }
                    }
                    n2757 = local write "1 6"(w3529) -> ()
                    n2758 = local write "1 7"(w3529) -> ()
                    n2759 = local write "1 8"(w3529) -> ()
                    n2760 = local write "1 9"(w3529) -> ()
                    n2761 = local write "1 10"(w3529) -> ()
                    n2762 = local write "1 12"(w3529) -> ()
                  }
                  frame #1 {
                    w3562 = FALSE ("流控帧")
                    w3563 = TRUE ("流控帧 2")
                    n2763 = global read "EV05全局变量1.vi" "授权功能"() -> (w3566:bool)
                    n2764 = case shown="假" w3566 {
                      tunnel: [TRUE ("发送成功") w3578] -> w3567
                      frame False {
                      }
                      frame True {
                        n2765 = local read "设备索引号"() -> (w3572:u16)
                        n2766 = local read "CAN卡类型"() -> (w3573:u32)
                        n2767 = local read "CAN端口"() -> (w3571:u16)
                        n2768 = call "标定授权发送.vi"("CAN卡类型"=w3573, "解锁类型"=enum16{"读取", "写", "下载"}."读取", "设备索引号"=w3572, "CAN端口"=w3571, "是否连接"=TRUE, "板选择"=0, "FUNC"=u32 1) -> ("发送成功"=w3578:bool)  [unwired: 8 out]
                      }
                    }
                    n2769 = case shown="真" w3567 {
                      tunnel: w3565 -> [w3580 w3581]
                      tunnel: w3564 -> [w3579 w3584]
                      tunnel: [w3580 w3586] -> w3569
                      tunnel: [w3579 w3585] -> w3568
                      frame False {
                      }
                      frame True {
                        n2770 = Flush Queue(queue=w3581, error in (no error)=w3584) -> (queue out=w3582:refnum<queue>, error out=w3583:errorcluster)  [unwired: 1 out]
                        n2771 = Enqueue Element(queue=w3582, element="全部读取" ("元素"), error in (no error)=w3583) -> (queue out=w3586:refnum<queue>, error out=w3585:errorcluster)  [unwired: 2 out]
                      }
                    }
                    n2772 = global write "EV05全局变量1.vi" "写入超时"(w3562) -> ()
                    n2773 = global write "EV05全局变量1.vi" "流控帧"(w3562) -> ()
                    n2774 = local write "写?"(w3562) -> ()
                    n2775 = local write "消除"(w3563) -> ()
                    n2776 = local write "控制1"(w3563) -> ()
                    n2777 = global write "EV05全局变量1.vi" "流控帧 2"(w3563) -> ()
                  }
                }
              }
            }
          }
          event "开启均衡": Value Change {
            n2778 = event-data() -> ("NewVal"=w3592:bool)  [unwired: 5 out]
            n2779 = case shown="真" w3592 {
              tunnel: w3591 -> [w3594 w3601]
              tunnel: w3590 -> [w3593 w3600]
              tunnel: [w3594 w3599] -> w3589
              tunnel: [w3593 w3598] -> w3588
              frame False {
              }
              frame True {
                n2780 = global read "EV05全局变量1.vi" "授权功能"() -> (w3596:bool)
                n2781 = case shown="假" w3596 {
                  tunnel: [TRUE ("发送成功") w3611] -> w3597
                  frame False {
                  }
                  frame True {
                    n2782 = local read "主从选择"() -> (w3603:enum32{"主板", "从板"})
                    n2783 = case shown="\"从板\"" w3603 {
                      tunnel: [0.0 ("FUNC") w3613] -> w3604
                      frame "主板", Default {
                      }
                      frame "从板" {
                        n2784 = local read "从板号"() -> (w3613:u8)
                      }
                    }
                    n2785 = local read "设备索引号"() -> (w3606:u16)
                    n2786 = local read "CAN卡类型"() -> (w3607:u32)
                    n2787 = local read "CAN端口"() -> (w3605:u16)
                    n2788 = call "标定授权发送.vi"("CAN卡类型"=w3607, "解锁类型"=enum16{"读取", "写", "下载"}."写", "设备索引号"=w3606, "CAN端口"=w3605, "是否连接"=TRUE, "板选择"=0, "FUNC"=w3604) -> ("发送成功"=w3611:bool)  [unwired: 8 out]
                  }
                }
                n2789 = case shown="真" w3597 {
                  tunnel: w3601 -> [w3615 w3620]
                  tunnel: w3600 -> [w3614 w3619]
                  tunnel: [w3615 w3617] -> w3599
                  tunnel: [w3614 w3616] -> w3598
                  frame False {
                  }
                  frame True {
                    n2790 = Enqueue Element(queue=w3620, element="开启均衡" ("元素"), error in (no error)=w3619) -> (queue out=w3617:refnum<queue>, error out=w3616:errorcluster)  [unwired: 2 out]
                  }
                }
                n2791 = call <vilib>:"Set Busy.vi"("disable click? (T)"=TRUE) -> ()  [unwired: 3 in, 8 out]
              }
            }
          }
          event "关闭均衡": Value Change {
            n2792 = event-data() -> ("NewVal"=w3625:bool)  [unwired: 5 out]
            n2793 = case shown="真" w3625 {
              tunnel: w3624 -> [w3627 w3634]
              tunnel: w3623 -> [w3626 w3633]
              tunnel: [w3627 w3632] -> w3622
              tunnel: [w3626 w3631] -> w3621
              frame False {
              }
              frame True {
                n2794 = global read "EV05全局变量1.vi" "授权功能"() -> (w3629:bool)
                n2795 = case shown="假" w3629 {
                  tunnel: [TRUE ("发送成功") w3644] -> w3630
                  frame False {
                  }
                  frame True {
                    n2796 = local read "主从选择"() -> (w3636:enum32{"主板", "从板"})
                    n2797 = case shown="\"从板\"" w3636 {
                      tunnel: [0.0 ("FUNC") w3646] -> w3637
                      frame "主板", Default {
                      }
                      frame "从板" {
                        n2798 = local read "从板号"() -> (w3646:u8)
                      }
                    }
                    n2799 = local read "设备索引号"() -> (w3639:u16)
                    n2800 = local read "CAN卡类型"() -> (w3640:u32)
                    n2801 = local read "CAN端口"() -> (w3638:u16)
                    n2802 = call "标定授权发送.vi"("CAN卡类型"=w3640, "解锁类型"=enum16{"读取", "写", "下载"}."写", "设备索引号"=w3639, "CAN端口"=w3638, "是否连接"=TRUE, "板选择"=0, "FUNC"=w3637) -> ("发送成功"=w3644:bool)  [unwired: 8 out]
                  }
                }
                n2803 = case shown="真" w3630 {
                  tunnel: w3634 -> [w3648 w3653]
                  tunnel: w3633 -> [w3647 w3652]
                  tunnel: [w3648 w3650] -> w3632
                  tunnel: [w3647 w3649] -> w3631
                  frame False {
                  }
                  frame True {
                    n2804 = Enqueue Element(queue=w3653, element="关闭均衡" ("元素"), error in (no error)=w3652) -> (queue out=w3650:refnum<queue>, error out=w3649:errorcluster)  [unwired: 2 out]
                  }
                }
                n2805 = call <vilib>:"Set Busy.vi"("disable click? (T)"=TRUE) -> ()  [unwired: 3 in, 8 out]
              }
            }
          }
          event "强制开启均衡": Value Change {
            n2806 = event-data() -> ("NewVal"=w3658:bool)  [unwired: 5 out]
            n2807 = case shown="真" w3658 {
              tunnel: w3657 -> [w3660 w3667]
              tunnel: w3656 -> [w3659 w3666]
              tunnel: [w3660 w3665] -> w3655
              tunnel: [w3659 w3664] -> w3654
              frame False {
              }
              frame True {
                n2808 = global read "EV05全局变量1.vi" "授权功能"() -> (w3662:bool)
                n2809 = case shown="假" w3662 {
                  tunnel: [TRUE ("发送成功") w3677] -> w3663
                  frame False {
                  }
                  frame True {
                    n2810 = local read "主从选择"() -> (w3669:enum32{"主板", "从板"})
                    n2811 = case shown="\"从板\"" w3669 {
                      tunnel: [0.0 ("FUNC") w3679] -> w3670
                      frame "主板", Default {
                      }
                      frame "从板" {
                        n2812 = local read "从板号"() -> (w3679:u8)
                      }
                    }
                    n2813 = local read "设备索引号"() -> (w3672:u16)
                    n2814 = local read "CAN卡类型"() -> (w3673:u32)
                    n2815 = local read "CAN端口"() -> (w3671:u16)
                    n2816 = call "标定授权发送.vi"("CAN卡类型"=w3673, "解锁类型"=enum16{"读取", "写", "下载"}."写", "设备索引号"=w3672, "CAN端口"=w3671, "是否连接"=TRUE, "板选择"=0, "FUNC"=w3670) -> ("发送成功"=w3677:bool)  [unwired: 8 out]
                  }
                }
                n2817 = case shown="真" w3663 {
                  tunnel: w3667 -> [w3681 w3686]
                  tunnel: w3666 -> [w3680 w3685]
                  tunnel: [w3681 w3683] -> w3665
                  tunnel: [w3680 w3682] -> w3664
                  frame False {
                  }
                  frame True {
                    n2818 = Enqueue Element(queue=w3686, element="强制均衡" ("元素"), error in (no error)=w3685) -> (queue out=w3683:refnum<queue>, error out=w3682:errorcluster)  [unwired: 2 out]
                  }
                }
                n2819 = call <vilib>:"Set Busy.vi"("disable click? (T)"=TRUE) -> ()  [unwired: 3 in, 8 out]
              }
            }
          }
